vi "VAH_plugin.vi"(9 "FPS":u32=20000, 10 "Frame counter":i32=333, 11 "Main Graph":dynamicdata(graph)=[{"t0"=timestamp(0 s since 1904-01-01), "dt"=1.0, "Y"=array[10000 elements], "attributes"=variant("NI_ChannelName"=variant(string "Voltage"), "NI_ExpIsRelativeTime"=variant(bool TRUE), "NI_ExpStartTimeStamp"=variant(timestamp timestamp(3710244565.071289 s since 1904-01-01)), "NI_ExpTimeStamp"=variant(timestamp timestamp(0 s since 1904-01-01)), "NI_ExpXDimension"=variant(string "t"))}, {"t0"=timestamp(0 s since 1904-01-01), "dt"=1.0, "Y"=array[10000 elements], "attributes"=variant("NI_ChannelName"=variant(string "Current"), "NI_ExpIsRelativeTime"=variant(bool TRUE), "NI_ExpStartTimeStamp"=variant(timestamp timestamp(3710244565.071289 s since 1904-01-01)), "NI_ExpTimeStamp"=variant(timestamp timestamp(0 s since 1904-01-01)), "NI_ExpXDimension"=variant(string "t"))}]) -> ()   [LabVIEW 2012]
panel:
  in  "Plot":bool=TRUE
  in  "Grid":bool=TRUE
  in  "Stop frame":i32=4000
  in  "Start frame":i32
  out "Active frame":i32
  in  "Line weight":u8=1
  in  "Cursor Color":u32(colorbox)=16711680
  in  "Graph Color":u32(colorbox)=16860
  in  "Y Cursor":bool=TRUE
  in  "X Cursor":bool=TRUE
  in  "Y Scale":bool=TRUE
  in  "X Scale":bool=TRUE
  out "Graph":cluster{"Y":dbl[], "Y":dbl[]}(graph)
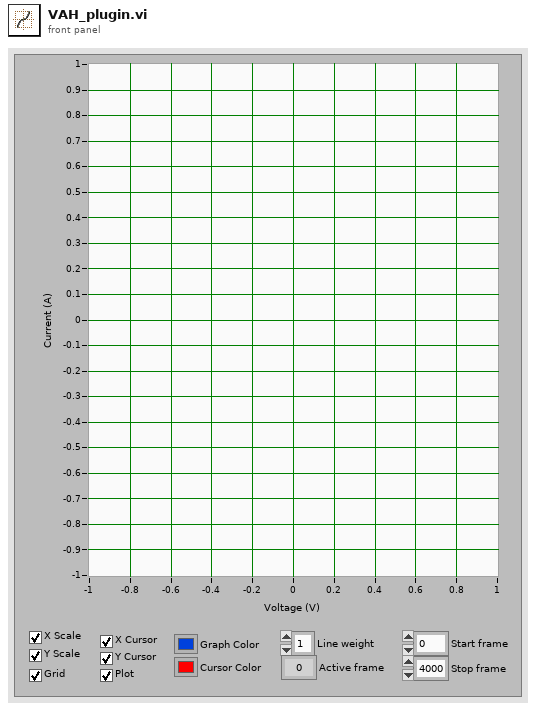
[diagram p1: front panel]
types:
  T1 = cluster{"Name":string, "Color":u32, "Style":u8, "Point Style":u8, "Name Visible":bool, "Allow Drag":bool, "Annotation Mode":u32, "Plot":i32, "Index":i32, "Position":cluster{"X":dbl, "Y":dbl}, "X Scale":u32, "Y Scale":u32, "Show Arrow":bool, "Lock Name":bool, "Plot Area":i32, "Label Offset":cluster{"X":dbl, "Y":dbl}}
  T2 = typedef "Video_analizer_settings.ctl" = cluster{"Current_shift":dbl, "Video_shift":dbl, "CurrentY_offset":dbl, "VoltageY_offset":dbl, "FIR_enable":bool, "Cutof_freq":dbl, "Order":u32}
  T3 = cluster{"Name":string, "Color":u32, "Style":u8, "Point Style":u8, "Name Visible":bool, "Allow Drag":bool, "Annotation Mode":u32, "Plot":i32, "Index":i32, "Position":cluster{"X":dbl, "Y":dbl}, "X Scale":u32, "Y Scale":u32, "Show Arrow":bool, "Lock Name":bool, "Plot Area":i32, "Label Offset":cluster{"X":dbl, "Y":dbl}}[]
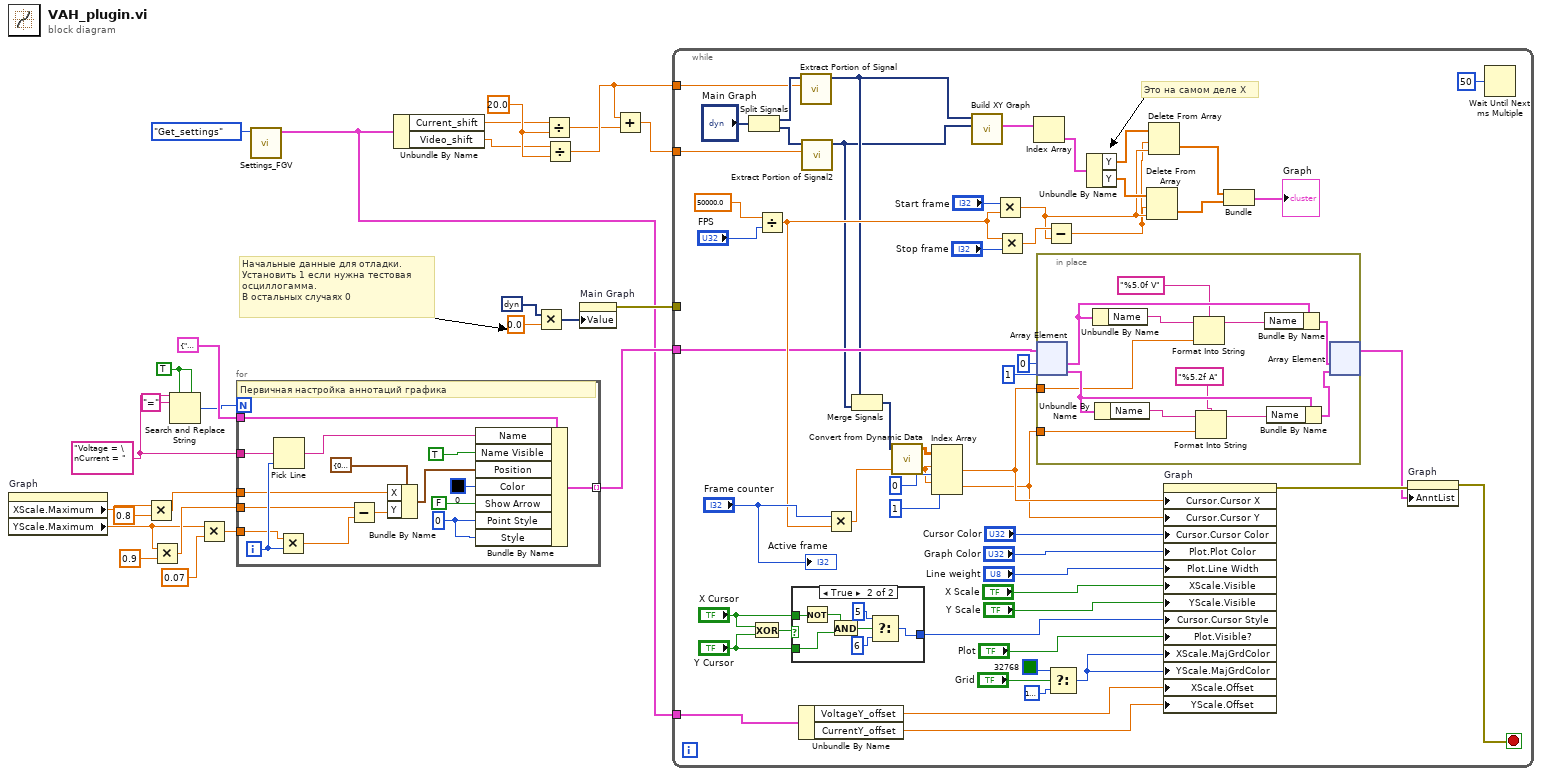
[diagram p0: block diagram]
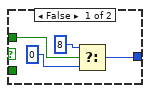
[diagram p2: hidden frame]
diagram:
  w15 = 20.0 ("y")
  w17 = TRUE ("multiline? (F)")
  w20 = "Voltage = \nCurrent = " ("multi-line string")
  # "Начальные данные для отладки. \nУстановить 1 если нужна тестовая \nосциллогамма.\nВ остальных случаях 0"
  n1 = property on="Graph" class="XYGraph (strict)"() -> ("XScale.Maximum"=w14:dbl, "YScale.Maximum"=w10:dbl)  [unwired: 2 in, 2 out]
  n2 = Multiply(x=w14, y=0.8) -> (x*y=w12:dbl)
  n3 = Multiply(x=w10, y=0.9) -> (x*y=w11:dbl)
  n4 = Search and Replace String(replace all?=w17, multiline?=w17, input string=w20, search string="=") -> (number of replacements=w21:i32)  [unwired: 4 in, 3 out]
  n5 = Multiply(x=w10, y=0.07) -> (x*y=w8:dbl)
  n6 = for {
    N: w21 -> [_]
    tunnel: T1 {"Name"="", "Color"=0, "Style"=0, "Point Style"=0, "Name Visible"=FALSE, "Allow Drag"=FALSE, "Annotation Mode"=0, "Plot"=0, "Index"=0, "Position"={"X"=0.0, "Y"=0.0}, "X Scale"=0, "Y Scale"=0, "Show Arrow"=FALSE, "Lock Name"=FALSE, "Plot Area"=0, "Label Offset"={"X"=0.0, "Y"=0.0}} ("element") -> [w39]
    tunnel: [w38] -> w18 mode=indexing
    tunnel: w20 -> [w37]
    tunnel: w12 -> [w31]
    tunnel: w11 -> [w29]
    tunnel: w8 -> [w27]
    i -> [w32]
    w35 = u8 0 ("Annotation Mode")
    # "Первичная настройка аннотаций графика"
    n7 = Pick Line(multi-line string=w37, line index=w32) -> (output string=w36:string)  [unwired: 1 in]
    n8 = Multiply(x=w27, y=w32) -> (x*y=w28:dbl)
    n9 = Subtract(x=w29, y=w28) -> (x-y=w30:dbl)
    n10 = Bundle By Name(cluster=cluster{"X":dbl, "Y":dbl} {"X"=0.0, "Y"=0.0} ("Position"), "X"=w31, "Y"=w30) -> (w33:cluster{"X":dbl, "Y":dbl})
    n11 = Bundle By Name(cluster=w39, "Name"=w36, "Name Visible"=TRUE, "Position"=w33, "Color"=u32 0, "Show Arrow"=FALSE, "Point Style"=w35, "Style"=w35) -> (w38:T1)
  }
  n12 = call "Settings_FGV.vi"("State"=enum16{"Get_settings", "Set_settings"}."Get_settings") -> ("Settings"=w1:T2)  [unwired: 9 in, 1 out]
  n13 = Unbundle By Name(w1) -> ("Current_shift"=w6:dbl, "Video_shift"=w5:dbl)
  n14 = Multiply(x=dynamicdata [{"t0"=timestamp(0 s since 1904-01-01), "dt"=1.0, "Y"=array[10000 elements], "attributes"=variant("NI_ChannelName"=variant(string "Voltage"), "NI_ExpIsRelativeTime"=variant(bool TRUE), "NI_ExpStartTimeStamp"=variant(timestamp timestamp(3710244565.071289 s since 1904-01-01)), "NI_ExpTimeStamp"=variant(timestamp timestamp(0 s since 1904-01-01)), "NI_ExpXDimension"=variant(string "t"))}, {"t0"=timestamp(0 s since 1904-01-01), "dt"=1.0, "Y"=array[10000 elements], "attributes"=variant("NI_ChannelName"=variant(string "Current"), "NI_ExpIsRelativeTime"=variant(bool TRUE), "NI_ExpStartTimeStamp"=variant(timestamp timestamp(3710244565.071289 s since 1904-01-01)), "NI_ExpTimeStamp"=variant(timestamp timestamp(0 s since 1904-01-01)), "NI_ExpXDimension"=variant(string "t"))}] ("Main Graph"), y=0.0) -> (x*y=w24:dynamicdata)
  n15 = Divide(x=w6, y=w15) -> (x/y=w3:dbl)
  n16 = Divide(x=w5, y=w15) -> (x/y=w4:dbl)
  n17 = property on="Main Graph" class="WFGraph (strict)"("Value"=w24) -> (error out=w26:errorcluster)  [unwired: 2 in, 1 out]
  n18 = Add(x=w4, y=w3) -> (x+y=w2:dbl)
  n19 = while {
    tunnel: w26 -> [_]
    tunnel: w18 -> [w59]
    tunnel: w4 -> [w50]
    tunnel: w2 -> [w49]
    tunnel: w1 -> [w45]
    stop <- w64 stop-if-true
    # "Это на самом деле Х"
    n20 = Split Signals("Main Graph") -> (w51:dynamicdata, w52:dynamicdata)  [unwired: 2 in]
    n21 = Exclusive Or(1:"Y Cursor", 2:"X Cursor") -> (0:w81:bool)
    n22 = Divide(x=50000.0, y="FPS") -> (x/y=w70:dbl)
    n23 = case shown="True" w81 {
      tunnel: "Y Cursor" -> [_ w117]
      tunnel: "X Cursor" -> [w109 w119]
      tunnel: [w110 w114] -> w80
      frame False {
        n24 = Select(t=u8 8, s=w109, f=u8 0) -> (s? t:f=w110:u8)
      }
      frame True {
        n25 = Not(x=w119) -> (.not. x?=w118:bool)
        n26 = And(x=w118, y=w117) -> (x .and. y?=w116:bool)
        n27 = Select(t=u8 5, s=w116, f=u8 6) -> (s? t:f=w114:u8)
      }
    }
    n28 = Unbundle By Name(w45) -> ("VoltageY_offset"=w44:dbl, "CurrentY_offset"=w43:dbl)
    n29 = call "Extract Portion of Signal"("Begin Sample"=w50, "Signals"=w51) -> ("Section"=w47:dynamicdata)  [unwired: 8 in, 1 out]
    n30 = call "Extract Portion of Signal2"("Begin Sample"=w49, "Signals"=w52) -> ("Section"=w46:dynamicdata)  [unwired: 8 in, 1 out]
    n31 = Multiply(x="Frame counter", y=w70) -> (x*y=w89:dbl)
    n32 = Merge Signals(w47, w46) -> (w48:dynamicdata)
    n33 = call "Convert from Dynamic Data"("Dynamic Data Type"=w48) -> ("Array"=w95:dbl[][])  [unwired: 3 in]
    n34 = Index Array(array=w95, index (row) #1=w89, index (col) #1=0 ("disabled index (col)"), index (row) #2=w89, index (col) #2=1 ("index (col)")) -> (element #1=w61:dbl, element #2=w60:dbl)
    n35 = call "Build XY Graph"("Y Input"=w46, "X Input"=w47) -> ("XY Graph"=w78:cluster{"Y":dbl[], "Y":dbl[]}[])  [unwired: 3 in, 6 out]
    n36 = Multiply(x="Start frame", y=w70) -> (x*y=w67:dbl)
    n37 = Multiply(x=w70, y="Stop frame") -> (x*y=w68:dbl)
    n38 = Index Array(array=w78) -> (element=w77:cluster{"Y":dbl[], "Y":dbl[]})  [unwired: 1 in]
    n39 = in-place {
      in-place-border: w61 -> [w100]
      in-place-border: w60 -> [w99]
      n40 = in-place-array #1(w59, 0, 1) -> (w107:T1, w102:T1)
      n41 = Unbundle By Name(w107) -> ("Name"=w108:string)
      n42 = Unbundle By Name(w102) -> ("Name"=w103:string)
      n43 = Format Into String(format string="%5.0f V", initial string=w108, w100) -> (resulting string=w106:string)  [unwired: 1 in, 1 out]
      n44 = Format Into String(format string="%5.2f A", initial string=w103, w99) -> (resulting string=w104:string)  [unwired: 1 in, 1 out]
      n45 = Bundle By Name(cluster=w107, "Name"=w106) -> (w105:T1)
      n46 = Bundle By Name(cluster=w102, "Name"=w104) -> (w101:T1)
      n47 = in-place-array #1(w105, w101) -> (w58:T3)  [unwired: 2 out]
    }
    n48 = Subtract(x=w68, y=w67) -> (x-y=w66:dbl)
    n49 = Select(t=u32 32768, s="Grid", f=u32 16777216) -> (s? t:f=w53:u32)
    n50 = Unbundle By Name(w77) -> ("Y"=w74:dbl[], "Y"=w75:dbl[])
    n51 = Delete From Array(array=w75, length=w66, index=w67) -> (deleted portion=w69:dbl[])  [unwired: 1 out]
    n52 = Delete From Array(array=w74, length=w66, index=w67) -> (deleted portion=w73:dbl[])  [unwired: 1 out]
    n53 = property on="Graph" class="XYGraph (strict)"("Cursor.Cursor X"=w61, "Cursor.Cursor Y"=w60, "Cursor.Cursor Color"="Cursor Color", "Plot.Plot Color"="Graph Color", "Plot.Line Width"="Line weight", "XScale.Visible"="X Scale", "YScale.Visible"="Y Scale", "Cursor.Cursor Style"=w80, "Plot.Visible?"="Plot", "XScale.MajGrdColor"=w53, "YScale.MajGrdColor"=w53, "XScale.Offset"=w44, "YScale.Offset"=w43) -> (error out=w65:errorcluster)  [unwired: 2 in, 1 out]
    n54 = Bundle("Y"=w73, "Y"=w69) -> (→"Graph":cluster{"Y":dbl[], "Y":dbl[]})  [unwired: 1 in]
    n55 = property on="Graph" class="XYGraph (strict)"(error in=w65, "AnntList"=w58) -> (error out=w64:errorcluster)  [unwired: 1 in, 1 out]
    n56 = Wait Until Next ms Multiple(millisecond multiple=u32 50) -> ()  [unwired: 1 out]
    "Active frame" <- "Frame counter"
  }
